vi "Generate Overlap SQL Query.vi"(8 "error in (no error)":errorcluster, 11 "Importing Transactions":refnum<class "Banking Statement.lvclass">) -> (0 "error out":errorcluster, 2 "Overlap Query":string, 3 "Overlapping Records":refnum<class "Statement.lvclass">)   [LabVIEW 2018, in "Banking Statement.lvclass"]
uses:
  Banking Statement.lvclass
  C:/Users/Jeff Tipps/Documents/Filthy-Lucre-Budgetizer/source/support/classes/Statement/Statement.lvclass
  Statement/Statement.lvclass
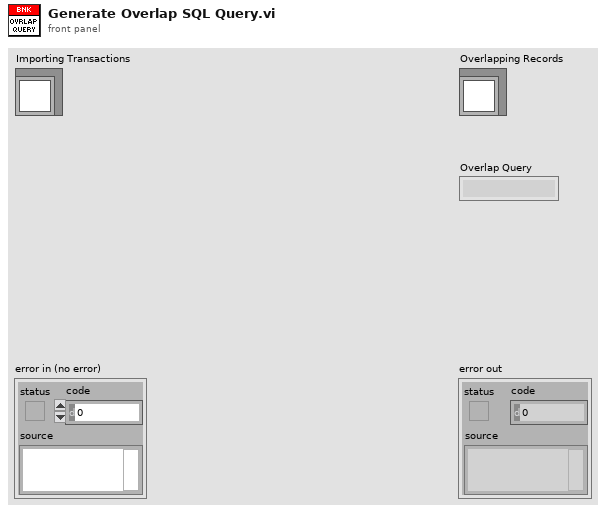
[diagram p1: front panel]
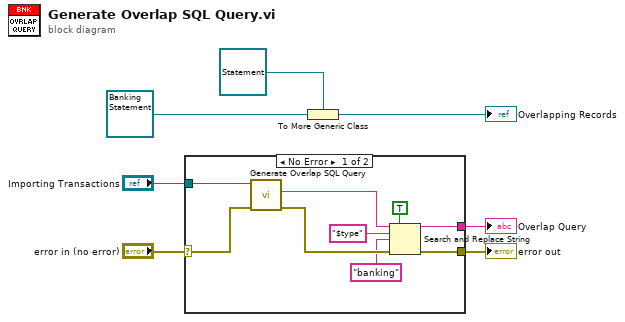
[diagram p0: block diagram]
diagram:
  n1 = case shown="No Error" "error in (no error)" {
    selector: "error in (no error)" -> [w9 w17]
    tunnel: "Importing Transactions" -> [w16 _]
    tunnel: [w11 w17] -> w6
    tunnel: [w10 _] -> w4
    frame No Error {
      n2 = call-parent "Generate Overlap SQL Query.vi"("error in (no error)"=w9, "Importing Transactions"=w16) -> ("error out"=w14:errorcluster, "Overlap Query"=w15:string)  [unwired: 7 in, 1 out]
      n3 = Search and Replace String(replace all?=TRUE ("replace all? (F)"), input string=w15, search string="$type", replace string="banking", error in=w14) -> (result string=w10:string, error out=w11:errorcluster)  [unwired: 3 in, 2 out]
    }
    frame Error {
    }
  }
  "error out" <- w6
  "Overlap Query" <- w4
  n4 = To More Generic Class(target class=refnum<class "Statement.lvclass"> refnum ("Overlapping Records"), reference=refnum<class "Banking Statement.lvclass"> refnum ("Banking Statement in")) -> (generic class reference=→"Overlapping Records":refnum<class "Statement.lvclass">)
